vi "Mutate.LVConfigFile.vi"() -> ()   [LabVIEW 2013, in "VeriStand Steps Version Mutation.lvlib"]
uses:
  VeriStand Steps Version Mutation.lvlib
  <vilib>/xml/Load XML File.vi
  <vilib>/xml/Close Reference(Node).vi
  <vilib>/xml/Close Reference(NNMap).vi
  <vilib>/xml/NI_XML.lvlib
  <resource>/objmgr/DOMUserDefRef.rc
  <vilib>/ni/Simple XML/Simple XML.lvlib
panel:
  out "error out":errorcluster
  in  "New VS Assembly Version":string="2013.0.0.0"
  in  "Old LV Config File Location":path=path "C:/Users/achurch/Documents/Source/XML Assembly Redirection Project/Examples XML Files/LabVIEW.exe.config" caption="Source TS ini File Location"
  in  "New TS Assembly Version":string="5.1.0.226"
  in  "New LV Config File Location":path=path "C:/Users/achurch/Documents/Source/XML Assembly Redirection Project/Examples XML Files/LabVIEW.exe.config_mod"
  # "Arguments:\n1: Old EXE Config File\n2: New EXE Config File\n3: New TS Assembly Version\n4: New VS Assembly Version"
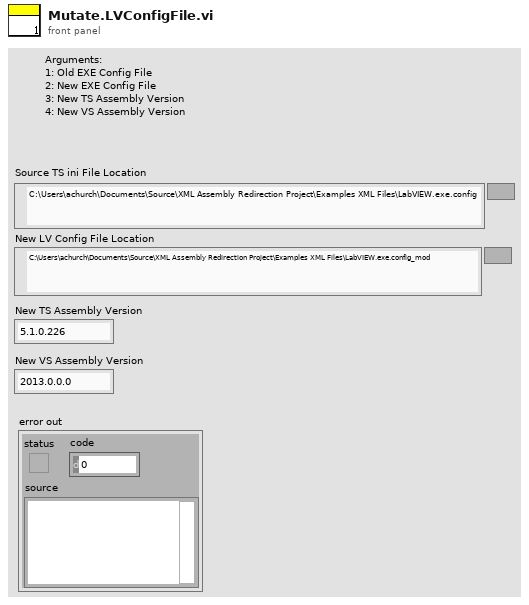
[diagram p1: front panel]
types:
  T1 = enum32{"invalid app kind", "Development System", "Run Time System", "Student Edition", "Embedded LabVIEW", "Evaluation", "Custom"}
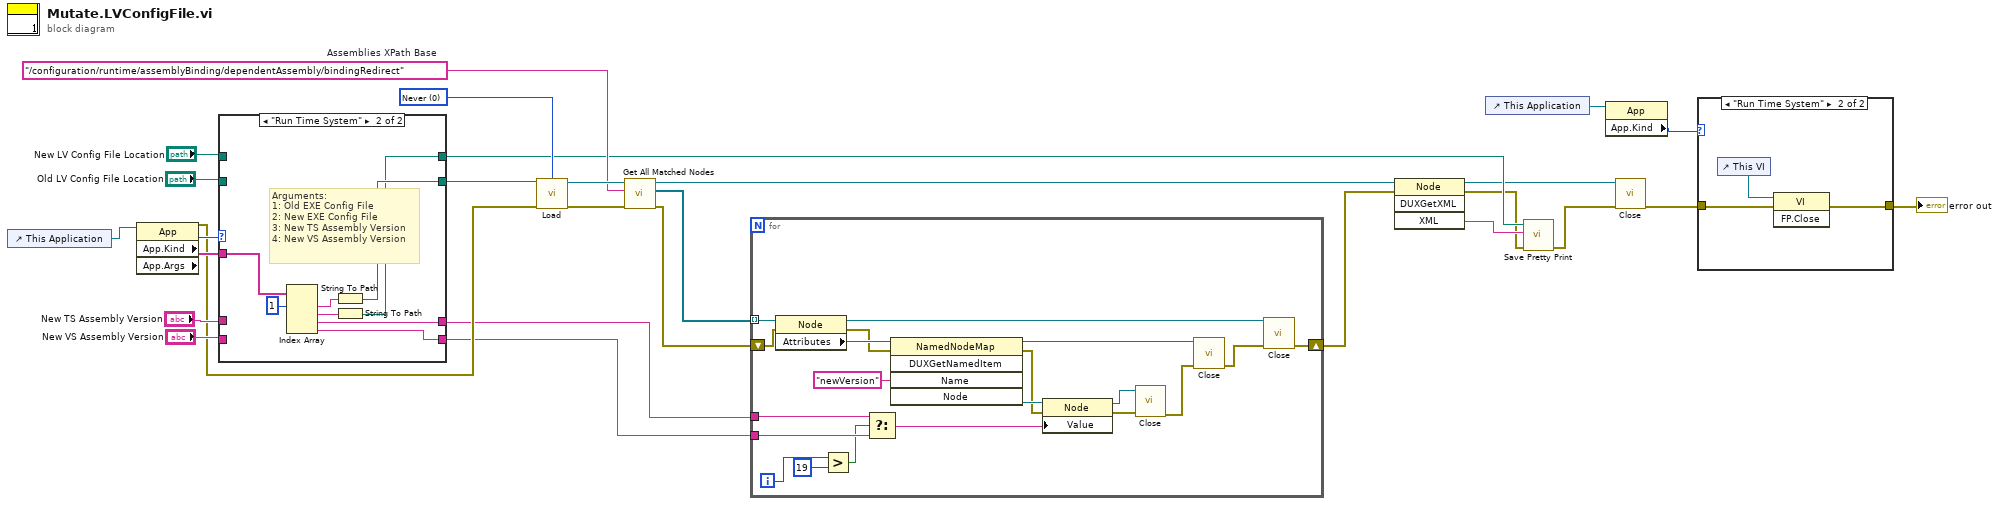
[diagram p0: block diagram]
diagram:
  w17 = "/configuration/runtime/assemblyBinding/dependentAssembly/bindingRedirect"  # Assemblies XPath Base
  w20 = 0 items=["Never", "Always", "Auto"] ("validate on load (Auto)")
  n1 = control-ref of="This Application"() -> (w6:refnum<vi>)
  n2 = property class="App"(reference=w6) -> (error out=w21:errorcluster, "App.Kind"=w27:T1, "App.Args"=w28:string[])  [unwired: 1 in, 1 out]
  n3 = case shown="\"Run Time System\"" w27 {
    tunnel: "New TS Assembly Version" -> [w30 _]
    tunnel: "New LV Config File Location" -> [w32 _]
    tunnel: "Old LV Config File Location" -> [w31 _]
    tunnel: w28 -> [_ w40]
    tunnel: [w32 w35] -> w10
    tunnel: [w31 w37] -> w22
    tunnel: [w30 w34] -> w14
    tunnel: "New VS Assembly Version" -> [w29 _]
    tunnel: [w29 w33] -> w5
    frame "Development System", Default {
    }
    frame "Run Time System" {
      # "Arguments:\n1: Old EXE Config File\n2: New EXE Config File\n3: New TS Assembly Version\n4: New VS Assembly Version"
      n4 = Index Array(array=w40, index #1=1 ("index")) -> (element #1=w38:string, element #2=w36:string, element #3=w34:string, element #4=w33:string)  [unwired: 3 in]
      n5 = String To Path(string=w38) -> (path=w37:path)
      n6 = String To Path(string=w36) -> (path=w35:path)
    }
  }
  n7 = call-poly <vilib>:"Load.vi"("path to XML document"=w22, "validate on load (Auto)"=w20, "error in (no error)"=w21) -> ("DOM document out"=w18:refnum<k20>, "error out"=w19:errorcluster)  [unwired: 10 in, 1 out]
  n8 = call <vilib>:"Get All Matched Nodes.vi"("error in (no error)"=w19, "XPath expression"=w17, "node in"=w18) -> ("error out"=w15:errorcluster, "node result array"=w16:refnum<k20>[], "node out"=w12:refnum<k20>)  [unwired: 6 in]
  n9 = for {
    tunnel: w16 -> [w60] mode=indexing
    tunnel: w14 -> [w46]
    shift-right: [w48] -> w13
    shift-left: w15 -> [w57]
    tunnel: w5 -> [w45]
    i -> [w44]
    n10 = property class="Node"(reference=w60, error in=w57) -> (reference out=w50:refnum<k20>, error out=w58:errorcluster, "Attributes"=w59:refnum<k20>)
    n11 = Greater?(x=w44, y=19) -> (0:w42:bool)
    n12 = Select(t=w46, s=w42, f=w45) -> (s? t:f=w41:string)
    n13 = invoke class="NamedNodeMap" method="DUXGetNamedItem"(reference=w59, error in=w58, "Name"="newVersion") -> (reference out=w52:refnum<k20>, error out=w55:errorcluster, "Node"=w56:refnum<k20>)  [unwired: 2 in, 2 out]
    n14 = property class="Node"(reference=w56, error in=w55, "Value"=w41) -> (reference out=w53:refnum<k20>, error out=w54:errorcluster)
    n15 = call-poly <vilib>:"Close.vi"("error in (no error)"=w54, "node"=w53) -> ("error out"=w51:errorcluster)  [unwired: 7 in]
    n16 = call-poly <vilib>:"Close.vi"("error in (no error)"=w51, "named node map"=w52) -> ("error out"=w49:errorcluster)  [unwired: 7 in]
    n17 = call-poly <vilib>:"Close.vi"("error in (no error)"=w49, "node"=w50) -> ("error out"=w48:errorcluster)  [unwired: 7 in]
  }
  n18 = invoke class="Node" method="DUXGetXML"(reference=w12, error in=w13) -> (reference out=w8:refnum<k20>, error out=w9:errorcluster, "XML"=w11:string)  [unwired: 2 in, 1 out]
  n19 = control-ref of="This Application"() -> (w3:refnum<vi>)
  n20 = call <vilib>:"Save Pretty Print.vi"("error in (no error)"=w9, "Pretty XML String"=w11, "XML file path"=w10) -> ("error out"=w7:errorcluster)  [unwired: 7 in, 1 out]
  n21 = property class="App"(reference=w3) -> ("App.Kind"=w4:T1)  [unwired: 1 in, 2 out]
  n22 = call-poly <vilib>:"Close.vi"("error in (no error)"=w7, "node"=w8) -> ("error out"=w2:errorcluster)  [unwired: 7 in]
  n23 = case shown="\"Run Time System\"" w4 {
    tunnel: w2 -> [w61 w63]
    tunnel: [w61 w62] -> w1
    frame "Development System", Default {
    }
    frame "Run Time System" {
      n24 = control-ref of="This VI"() -> (w64:refnum<vi>)
      n25 = invoke class="VI" method="FP.Close"(reference=w64, error in=w63) -> (error out=w62:errorcluster)  [unwired: 1 in, 2 out]
    }
  }
  "error out" <- w1
